vi "stopServerProcess.vi"(8 "error in (no error)":errorcluster, 11 "tcpServer in":refnum<class "TcpServer.lvclass">) -> (0 "error out":errorcluster, 3 "tcpServer out":refnum<class "TcpServer.lvclass">)   [LabVIEW 2018, in "TcpServer.lvclass"]
doc: "Send notification to stop a process running inside of runServer.vi."
uses:
  TcpServer.lvclass
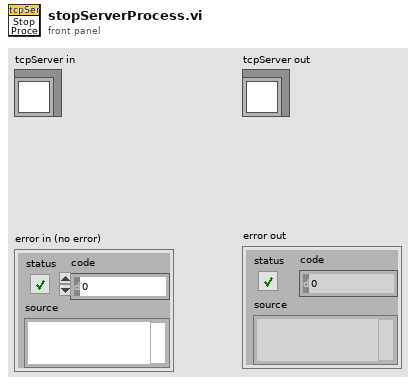
[diagram p1: front panel]
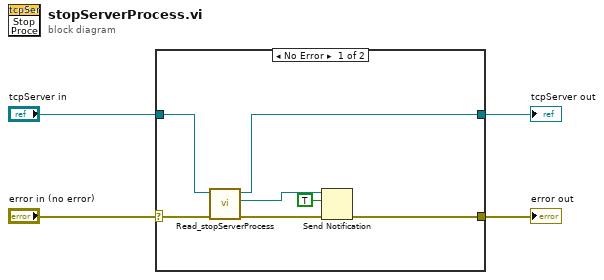
[diagram p0: block diagram]
diagram:
  n1 = case shown="No Error" "error in (no error)" {
    selector: "error in (no error)" -> [w10 w12]
    tunnel: [w11 w12] -> w3
    tunnel: "tcpServer in" -> [w8 w13]
    tunnel: [w7 w13] -> w1
    frame No Error {
      n2 = call-dynamic "Read_stopServerProcess.vi"("error in (no error)"=w10, "TcpServer in"=w8) -> ("error out"=w9:errorcluster, "stopServerProcess"=w6:refnum<notifier>, "TcpServer out"=w7:refnum<class "TcpServer.lvclass">)  [unwired: 7 in]
      n3 = Send Notification(notification=TRUE, notifier=w6, error in (no error)=w9) -> (error out=w11:errorcluster)  [unwired: 1 out]
    }
    frame Error {
    }
  }
  "error out" <- w3
  "tcpServer out" <- w1
